vi "Iniciar Adquisicion.vi"(8 "error in (no error)":errorcluster, 11 "Webcam in":refnum<class "Webcam.lvclass">) -> (0 "error out":errorcluster, 3 "Webcam out":refnum<class "Webcam.lvclass">)   [LabVIEW 2020, in "Webcam.lvclass"]
uses:
  Webcam.lvclass
  Abstracta/Camara/Camara.lvclass
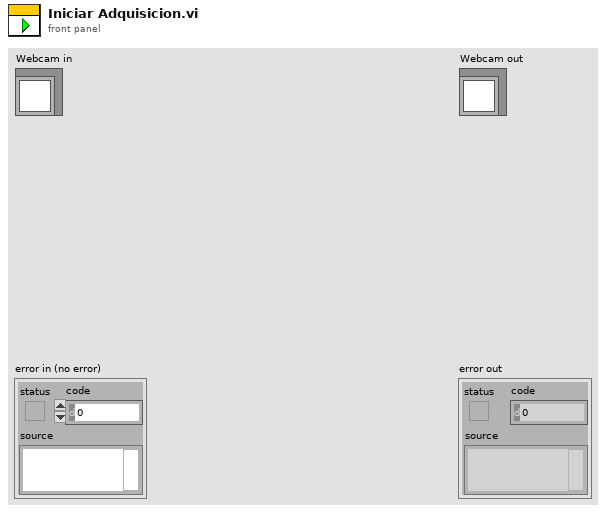
[diagram p1: front panel]
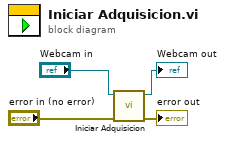
[diagram p0: block diagram]
diagram:
  n1 = call-parent "Iniciar Adquisicion.vi"("error in (no error)"="error in (no error)", "Camara in"="Webcam in") -> ("error out"=→"error out":errorcluster, "Camara out"=→"Webcam out":refnum<class "Webcam.lvclass">)  [unwired: 8 in]
